vi "testRegTcpServerUserEvent.vi"(8 "error in (no error)":errorcluster) -> (0 "error out":errorcluster)   [LabVIEW 2018]
doc: "Test the regTcpServerUserEvent.vi."
uses:
  src/TcpServerBase/TcpServerBase.lvclass
  src/TcpServerBase/TcpServerBase.lvclass/TcpServerBase.ctl
  <vilib>/addons/_JKI Toolkits/Caraya/classes/Assert/Assert Equal Type_Variant.vi
  <vilib>/addons/_JKI Toolkits/Caraya/classes/Test/Test.lvclass
  <vilib>/addons/_JKI Toolkits/Caraya/classes/Assert/Assert.lvclass
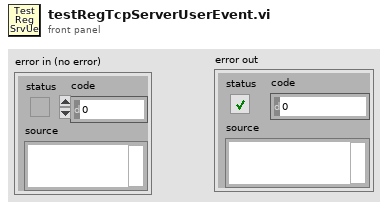
[diagram p1: front panel]
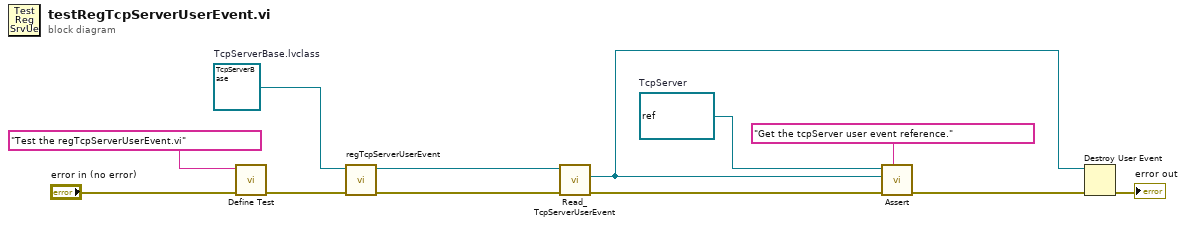
[diagram p0: block diagram]
diagram:
  w4 = refnum<user-event> refnum  # TcpServer
  w9 = refnum<class "TcpServerBase.lvclass"> refnum  # TcpServerBase.lvclass
  n1 = call <vilib>:"Define Test.vi"("error in (no error)"="error in (no error)", "Label (VI Title)"="Test the regTcpServerUserEvent.vi") -> ("error out"=w8:errorcluster)  [unwired: 9 in]
  n2 = call "regTcpServerUserEvent.vi"("error in (no error)"=w8, "tcpServerBase in"=w9) -> ("error out"=w7:errorcluster, "tcpServerBase out"=w6:refnum<class "TcpServerBase.lvclass">)  [unwired: 8 in]
  n3 = call "Read_TcpServerUserEvent.vi"("error in (no error)"=w7, "TcpServerBase in"=w6) -> ("error out"=w5:errorcluster, "TcpServer"=w1:refnum<user-event>)  [unwired: 7 in, 1 out]
  n4 = call-poly <vilib>:"Assert.vi"("Label"="Get the tcpServer user event reference.", "error in (no error)"=w5, "Y"=w1, "X"=w4) -> ("error out"=w3:errorcluster)  [unwired: 7 in]
  n5 = Destroy User Event(user event=w1, error in=w3) -> (error out=→"error out":errorcluster)
